vi "fgv_pc_cam_param.vi"(7 "cmd":enum16{"ini", "read", "write"}(ring), 11 "cam_param_in":T3={"adjust sat"=0, "edge detect param"={"Sigma"=1.0, "HThresh"=0.9, "LThres"=0.2, "WindowSize"=9}} {"edge detect param"."WindowSize" scale=0.0..10.0; "edge detect param"."LThres" min=0 max=1 scale=0.0..1.0; "edge detect param"."HThresh" min=0 max=1 scale=0.0..1.0; "edge detect param"."Sigma" min=0 max=1 scale=0.0..10.0; "adjust sat" scale=0.0..255.0}) -> (3 "cam_param_out":T2)   [LabVIEW 2018]
panel:
  in  "edge detect param":T1={"Sigma"=1.0, "HThresh"=0.9, "LThres"=0.2, "WindowSize"=9} {"LThres" min=0 max=1 format="%.2f"; "HThresh" min=0 max=1 format="%.2f"; "Sigma" min=0 max=1 format="%.2f"}
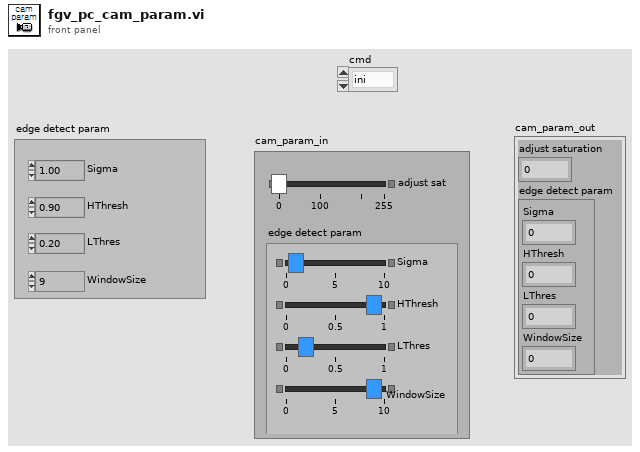
[diagram p1: front panel]
types:
  T1 = cluster{"Sigma":sgl, "HThresh":sgl, "LThres":sgl, "WindowSize":i32}
  T2 = cluster{"adjust saturation":u32, "edge detect param":cluster{"Sigma":sgl, "HThresh":sgl, "LThres":sgl, "WindowSize":i32}}
  T3 = cluster{"adjust sat":u32, "edge detect param":cluster{"Sigma":sgl, "HThresh":sgl, "LThres":sgl, "WindowSize":i32}}
  T4 = cluster{"adjust saturation level":u32, "edge detector parameters":cluster{"Sigma":sgl, "HThresh":sgl, "LThres":sgl, "WindowSize":i32}}
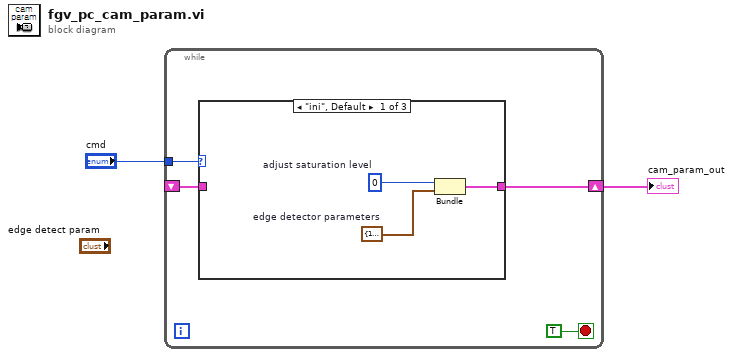
[diagram p0: block diagram]
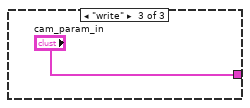
[diagram p3: hidden frame]
diagram:
  n1 = while {
    tunnel: "cmd" -> [w6]
    shift-right: [w4] -> w1
    shift-left: _ -> [w3]
    stop <- TRUE stop-if-true
    n2 = case shown="\"ini\", Default" w6 {
      tunnel: [w7 w10 "cam_param_in"] -> w4
      tunnel: w3 -> [_ w10 _]
      frame "ini", Default {
        w8 = u32 0  # adjust saturation level
        w9 = T1 {"Sigma"=1.0, "HThresh"=0.9, "LThres"=0.2, "WindowSize"=9}  # edge detector parameters
        n3 = Bundle("adjust saturation level"=w8, "edge detector parameters"=w9) -> (w7:T4)  [unwired: 1 in]
      }
      frame "read" {
      }
      frame "write" {
      }
    }
  }
  "cam_param_out" <- w1
